vi "Global Tags.vi"() -> ()   [LabVIEW 2016, in "RM.Shared.lvlib"]
uses:
  RM.Shared.lvlib
panel:
  in  "Tags":enum32{"Client", "Server"}(tab)=enum."Server"
  in  "Client":string="RM.Client"
  in  "Reservation Format String":string="RM.Reservation.%s"
  in  "Server":string="RM.Server"
  in  "Visualizer Status":string="rm.visualizer.status"
  in  "Reservation Info String":string="\n\nOwning CD \n%s\n\nResource Name\n%s\n\nInput Type\n%s\n\nDatatype\n%s\n\nNotes\n%s"
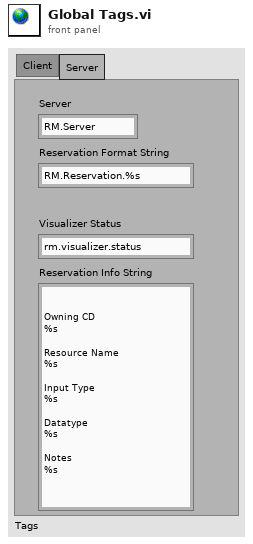
[diagram p1: front panel]
diagram:
